vi "Logger Queue FGV.vi"(7 "Read?":bool, 11 "LogReference Instance":refnum<class "LoggerReference.lvclass">) -> (3 "LogReference Instance Out":refnum<class "LoggerReference.lvclass">)   [LabVIEW 2018, in "MVA Framework.lvlib" / "Singleton Event Log.lvlib"]
doc: "--\nCopyright © 2017 Composed SystemsI All rights reserved.\n\nAuthor: Jon McBee <jon.mcbee@composed.io>\n\nThis library is provided \"AS IS\" ,WITHOUT WARRANTIES OR\nCONDITIONS OF ANY KIND, either express or implied.\n\nComposed Systems -- composed.io\n\nStream 0.0.1.1\nJon McBee - Composed Systems\nCopyright (c) 2017, Composed Systems"
uses:
  Singleton Event Log.lvlib
  LoggerReference/LoggerReference.lvclass
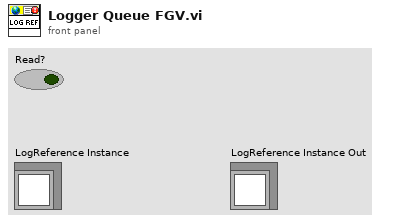
[diagram p1: front panel]
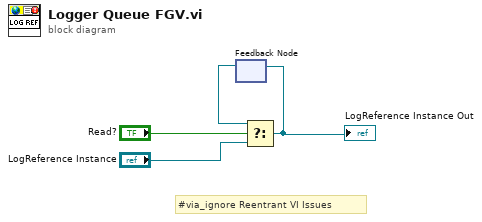
[diagram p0: block diagram]
diagram:
  # "#via_ignore Reentrant VI Issues"
  n1 = feedback #1() -> (w2:refnum<class "LoggerReference.lvclass">)  [unwired: 1 in]
  n2 = Select(t=w2, s="Read?", f="LogReference Instance") -> (s? t:f=w1:refnum<class "LoggerReference.lvclass">)
  "LogReference Instance Out" <- w1
  n3 = feedback-in #1(w1) -> ()
